vi "Fill all amplitude registers.vi"(11 "error in (no error)":errorcluster) -> (6 "String":string, 15 "error out":errorcluster)   [LabVIEW 2010]
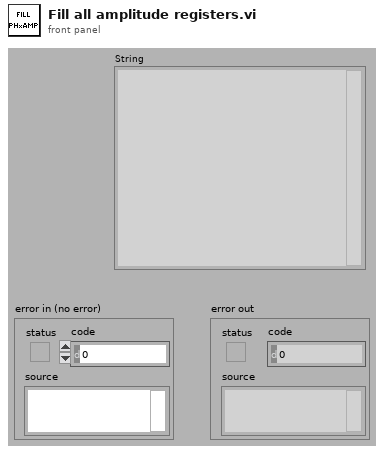
[diagram p1: front panel]
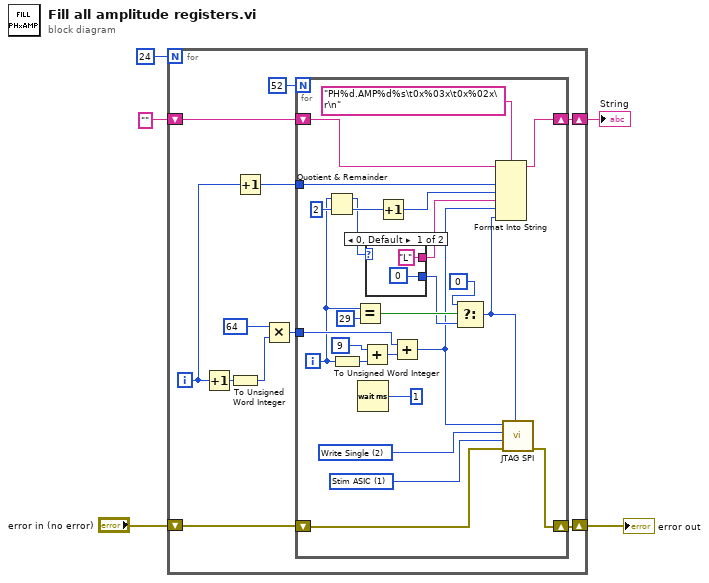
[diagram p0: block diagram]
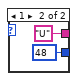
[diagram p2: hidden frame]
diagram:
  n1 = for {
    N: 24 -> [_]
    shift-right: [w14] -> w3
    shift-left: "" -> [w15]
    shift-right: [w8] -> w1
    shift-left: "error in (no error)" -> [w7]
    i -> [w10]
    n2 = Increment(x=w10) -> (x+1=w6:i32)
    n3 = To Unsigned Word Integer(number=w6) -> (unsigned 16bit integer=w12:u16)
    n4 = Increment(x=w10) -> (x+1=w9:i32)
    n5 = Multiply(x=u16 64, y=w12) -> (x*y=w11:u16)
    n6 = for {
      N: 52 -> [_]
      shift-right: [w35] -> w14
      shift-left: w15 -> [w36]
      tunnel: w11 -> [w38]
      tunnel: w9 -> [w34]
      shift-right: [w20] -> w8
      shift-left: w7 -> [w19]
      i -> [w29]
      w22 = u16 1 items=["Power ASIC", "Stim ASIC", "MICS Radio", "FRAM"] ("Target")
      w21 = u16 2 items=["Power UP", "Power DN", "Write Single", "Read Single", "Write Block", "Read Block", "Write Masked", "Test Value"] ("Function")
      n7 = Quotient & Remainder(x=w29, y=2) -> (x-y*floor(x/y)=w31:i32, floor(x/y)=w32:i32)
      n8 = To Unsigned Word Integer(number=w29) -> (unsigned 16bit integer=w41:u16)
      n9 = Equal?(x=w29, y=29) -> (x = y?=w27:bool)
      n10 = Wait (ms)(milliseconds to wait=u32 1) -> ()  [unwired: 1 out]
      n11 = Add(x=u16 9, y=w41) -> (x+y=w39:u16)
      n12 = case shown="0, Default" w31 {
        tunnel: ["L" "U"] -> w30
        tunnel: [u8 0 u8 48] -> w26
        frame 0, Default {
        }
        frame 1 {
        }
      }
      n13 = Increment(x=w32) -> (x+1=w24:i32)
      n14 = Add(x=w38, y=w39) -> (x+y=w17:u16)
      n15 = Select(t=u8 0, s=w27, f=w26) -> (s? t:f=w18:u8)
      n16 = Format Into String(format string="PH%d.AMP%d%s\t0x%03x\t0x%02x\r\n", initial string=w36, w34, w24, w30, w17, w18) -> (resulting string=w35:string)  [unwired: 1 in, 1 out]
      n17 = call "JTAG SPI.vi"("Value"=w18, "error in (no error)"=w19, "Target"=w22, "Function"=w21, "Address"=w17) -> ("error out"=w20:errorcluster)  [unwired: 3 in, 3 out]
    }
  }
  "String" <- w3
  "error out" <- w1
